vi "main.vi"() -> ()   [LabVIEW 2016]
uses:
  TypeDefs/scan_settings.ctl
  TypeDefs/State Enumerate Ring.ctl
panel:
  out "Settings folder path":path
  out "Date array":string[](array[string])
  out "Abort initalisation?":bool
  out "Scan stopped?":bool
  in  "Tab Control":T1(tab)
  in  "Manual mode":bool
  in  "Load details from file":bool
  in  "Save details to file":bool
  out "Keithley SMU":bool
  in  "User Name":string
  in  "Exeriment Title":string
  out "Status:":string
  in  "Device details":T2={"Cell Position"=1, "Cell Label"="", "Pixel to measure"=0, "Area (cm^2)"=0.0919, "Variable"="", "Variable value"="", "Scan settings"=0} {"Scan settings" items=["Default_inv"]; "Pixel to measure" items=["All", "1", "2", "3", "4", "5", "6", "7", "8"]}
  in  "Scan settings":T3={"J-V scan"=TRUE, "Start voltage (V)"=0.0, "End voltage (V)"=1.4, "Step voltage (V)"=0.01, "Scan both directions"=TRUE, "Inverted device structure"=FALSE, "Settling delay (ms)"=10.0, "Measurement speed"=0, "Scan rate (V/s)"=1.0, "Stabilisation time (s)"=0.0, "Stabilisation mode"=0, "Stabilisation value (V or A) "=0.0, "Illumination"=2, "Stabilisation in the dark?"=FALSE, "Repeat light scans"=FALSE, "No. of repeat scans"=2.0, "Only repeat for best pixel"=7, "J-t scan"=FALSE, "J-t best pixel only"=7, "J-t start voltage (V)"=0.0, "J-t end voltage (V)"=1.4, "J-t step voltage (V)"=0.01, "Step time (s)"=1.0, "J-t scan both directions"=TRUE, "J-t inverted device structure"=FALSE, "J-t settling delay (ms)"=0.0, "J-t measurement speed"=0, "J-t illumination"=1, "Max. power stabilisation"=FALSE, "Max power best pixel only"=7, "Max. power point tracker"=FALSE, "Vmp from J-V scan"=FALSE, "Max P stab. Specific voltage"=FALSE, "Vmp (V)"=0.7, "Stabilisation time step (s)"=1.0, "Total stabilisation time (s)"=100.0} {"J-t settling delay (ms)" min=10.0; "J-t illumination" items=["Light only", "Dark only", "Light then dark", "Dark then light"]; "Measurement speed" items=["Fast", "Normal", "High accuracy"]; "Illumination" items=["Light only", "Dark only", "Light then dark", "Dark then light"]; "Only repeat for best pixel" items=["only for best pixel", "for best 2 pixels", "for best 3 pixels", "for best 4 pixels", "for best 5 pixels", "for best 6 pixels", "for best 7 pixels", "for all pixels"]; "No. of repeat scans" min=1.0 step=1.0; "Max power best pixel only" items=["only the best pixel", "the best 2 pixels", "the best 3 pixels", "the best 4 pixels", "the best 5 pixels", "the best 6 pixels", "the best 7 pixels", "all pixels"]; "J-t best pixel only" items=["only the best pixel", "the best 2 pixels", "the best 3 pixels", "the best 4 pixels", "the best 5 pixels", "the best 6 pixels", "the best 7 pixels", "all pixels"]; "J-t measurement speed" items=["Fast", "Normal", "High Accuracy"]; "Stabilisation mode" items=["V", "I"]; "Settling delay (ms)" min=10.0}
  in  "Delete settings":bool
  in  "Save new settings":bool
  in  "Check Saved Settings":u16(ring) items=["Default_inv"]
  in  "Save New Settings As...":string
  in  "Update":bool
  in  "Exit":bool
  out "QuickMUX":bool
  in  "Lamp off":bool=TRUE
  out "Measurement status:":string
  out "Log Table":string[][](table)
  out "JV Curve":cluster{"Y":dbl[], "Y":dbl[]}[](graph)
  in  "Stop Scan 2":bool
  in  "Start Scan":bool
  in  "Generate report":bool
  out "Current (A)":dbl
  in  "Pixel":i64=1 min=1 max=8 step=1
  in  "error in (no error) 3":errorcluster
  in  "Change pin on pcb":bool
  in  "Measure current":bool
  out "File path for master log":path
  out "VISA resource name":refnum<visa-resource-name>="GPIB1::24::INSTR"
  # "Connected instruments"
  # "Label"
  # "Pixel"
  # "Condition"
  # "Jsc"
  # "Voc"
  # "PCE"
  # "FF"
  # "Vmp"
  # "Pixel Selection"
  # "Current Measurement"
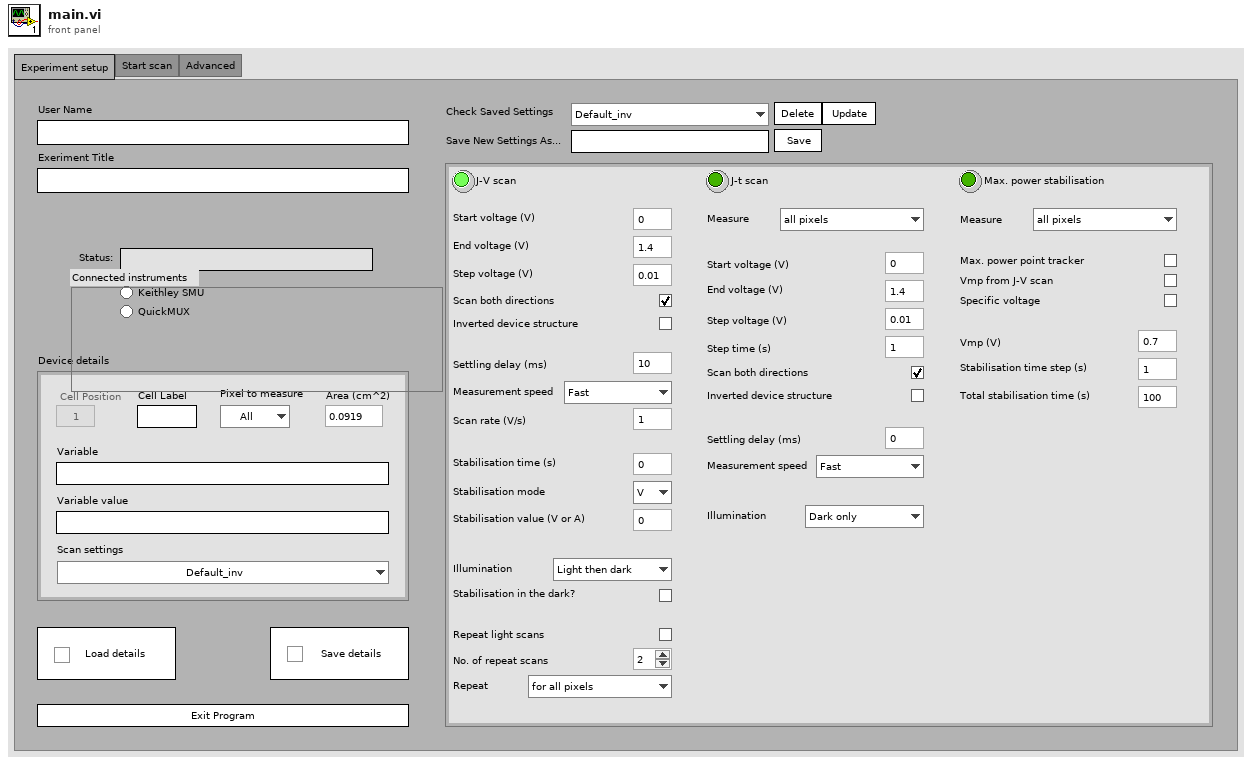
[diagram p1: front panel]
types:
  T1 = enum32{"Experiment setup", "Start scan", "Advanced"}
  T2 = cluster{"Cell Position":i32, "Cell Label":string, "Pixel to measure":u16, "Area (cm^2)":dbl, "Variable":string, "Variable value":string, "Scan settings":u16}
  T3 = typedef "scan_settings.ctl" = cluster{"J-V scan":bool, "Start voltage (V)":dbl, "End voltage (V)":dbl, "Step voltage (V)":dbl, "Scan both directions":bool, "Inverted device structure":bool, "Settling delay (ms)":dbl, "Measurement speed":u8, "Scan rate (V/s)":dbl, "Stabilisation time (s)":dbl, "Stabilisation mode":u16, "Stabilisation value (V or A) ":dbl, "Illumination":u16, "Stabilisation in the dark?":bool, "Repeat light scans":bool, "No. of repeat scans":dbl, "Only repeat for best pixel":u16, "J-t scan":bool, "J-t best pixel only":u16, "J-t start voltage (V)":dbl, "J-t end voltage (V)":dbl, "J-t step voltage (V)":dbl, "Step time (s)":dbl, "J-t scan both directions":bool, "J-t inverted device structure":bool, "J-t settling delay (ms)":dbl, "J-t measurement speed":u16, "J-t illumination":u16, "Max. power stabilisation":bool, "Max power best pixel only":u16, "Max. power point tracker":bool, "Vmp from J-V scan":bool, "Max P stab. Specific voltage":bool, "Vmp (V)":dbl, "Stabilisation time step (s)":dbl, "Total stabilisation time (s)":dbl}
  T4 = typedef "State Enumerate Ring.ctl" = enum16{"Initialise", "Idle", "Measure", "Notify"}
  T5 = enum8{"Enabled", "Disabled", "Disabled and Grayed Out"}
  T6 = cluster{"Cell Position":i32, "Cell Label":string, "Pixel to measure":u16, "Area (cm^2)":dbl, "Variable":string, "Variable value":string, "Scan settings in queue":u16, "Light or dark":string, "Measurement type":string}[]
  T7 = cluster{"Cell Position":i32, "Cell Label":string, "Pixel to measure":u16, "Area (cm^2)":dbl, "Variable":string, "Variable value":string, "Scan settings in queue":u16, "Light or dark":string, "Measurement type":string}
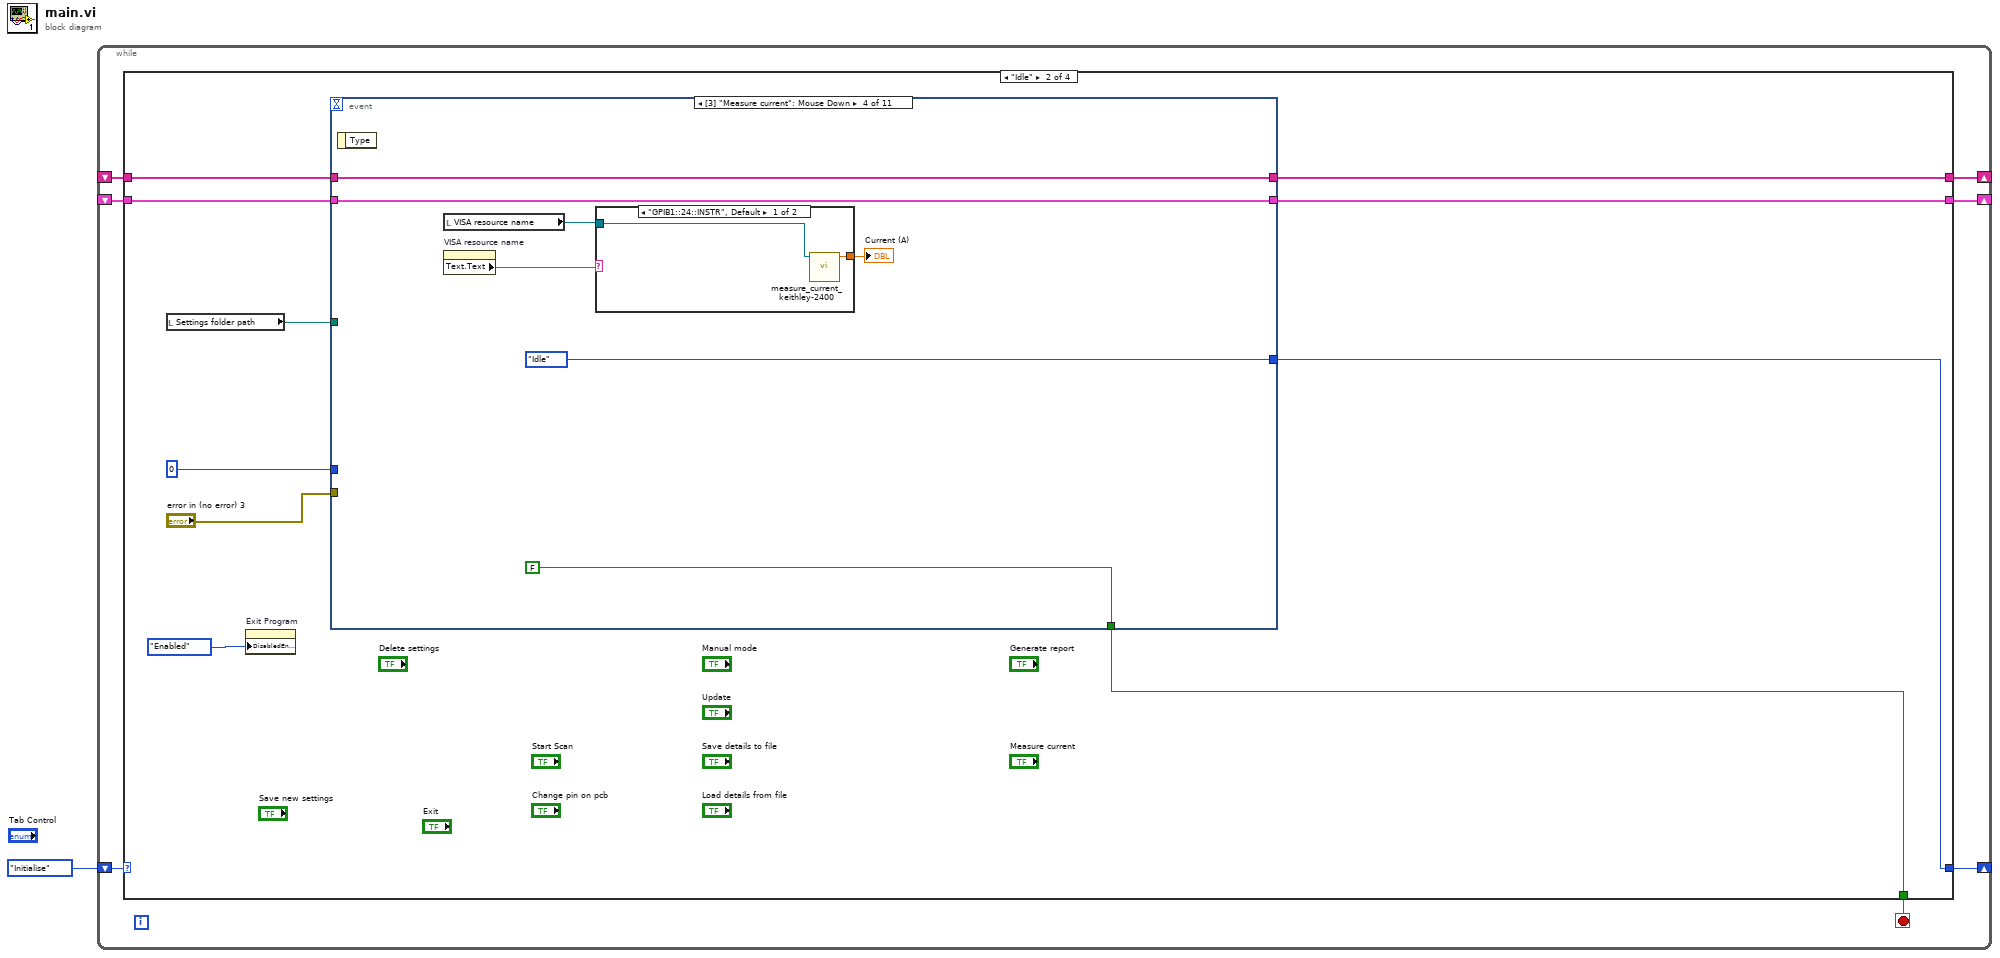
[diagram p0: block diagram]
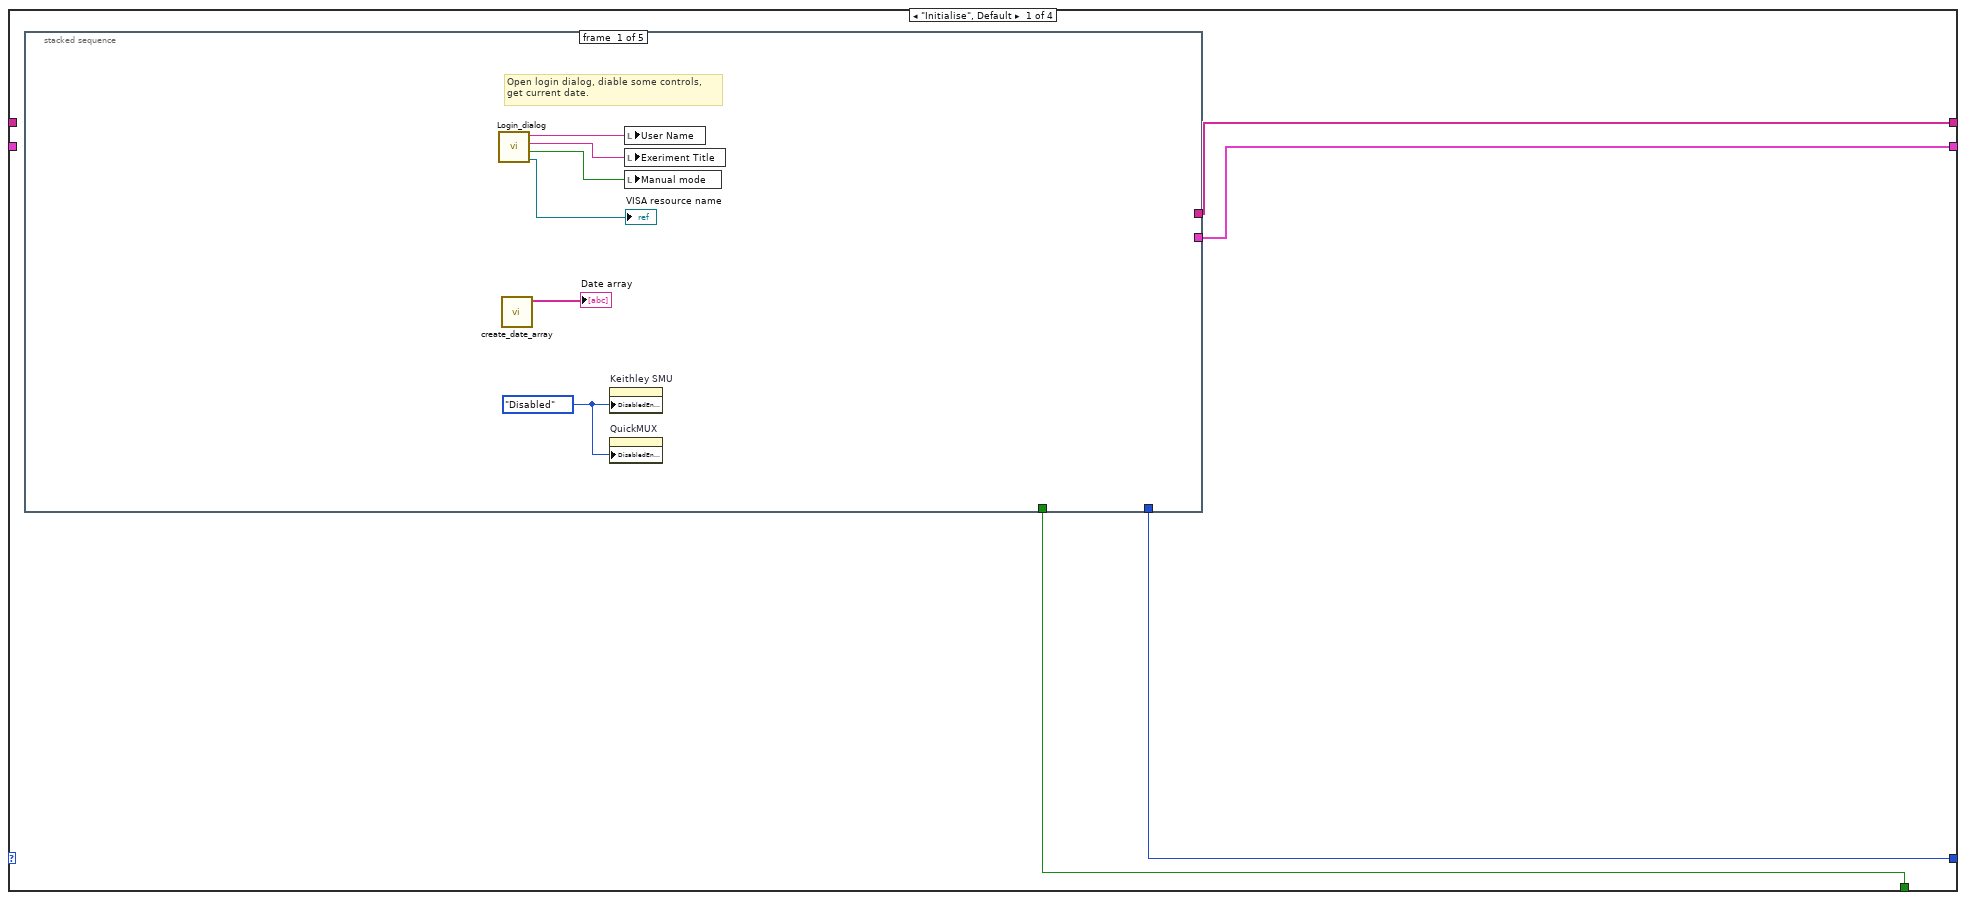
[diagram p2: hidden frame]
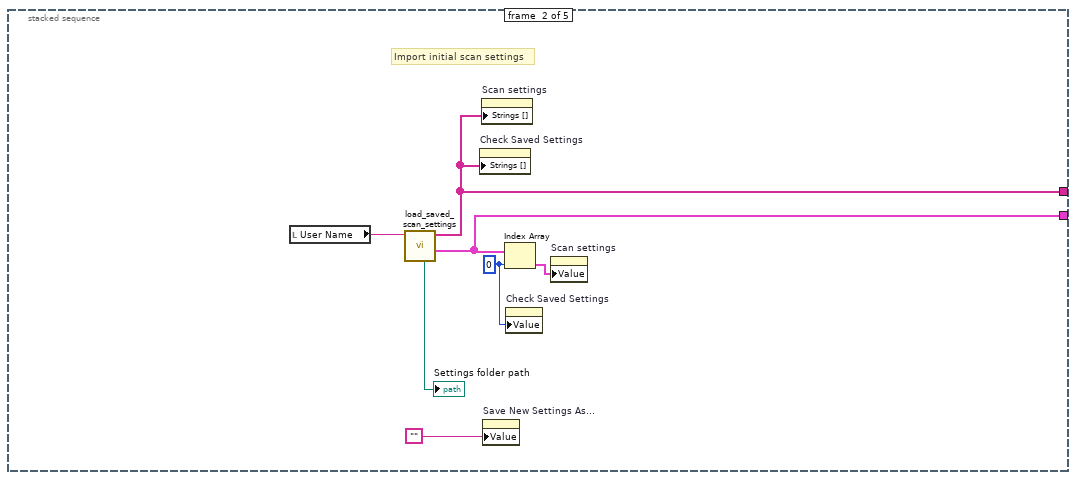
[diagram p3: hidden frame]
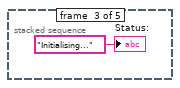
[diagram p4: hidden frame]
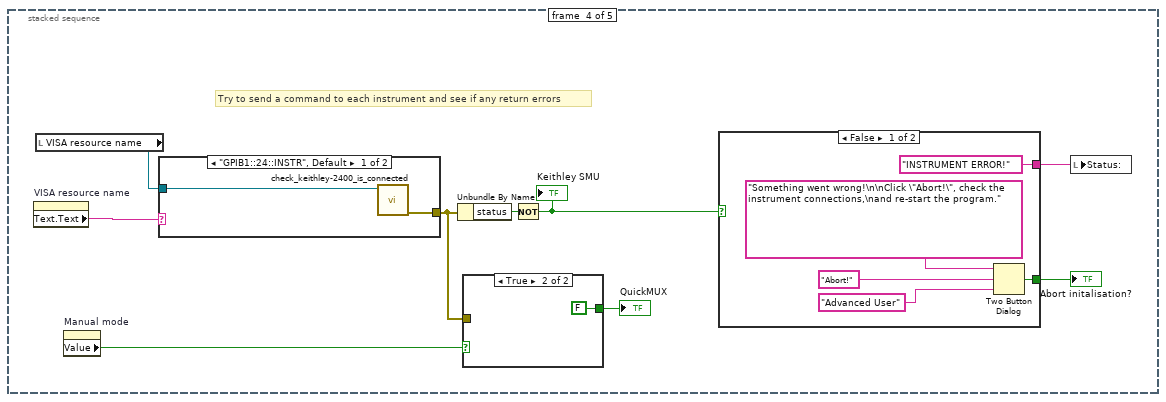
[diagram p5: hidden frame]
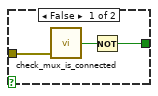
[diagram p6: hidden frame]
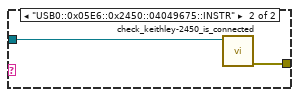
[diagram p7: hidden frame]
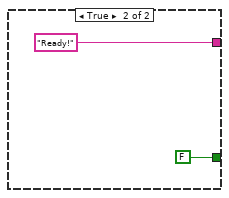
[diagram p8: hidden frame]
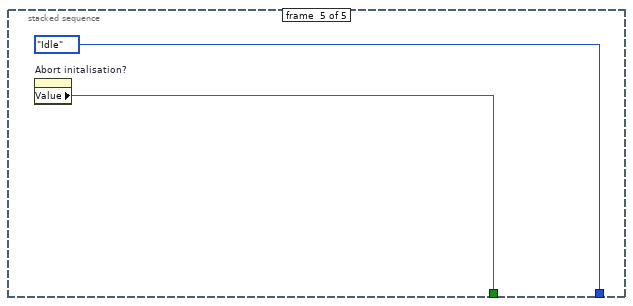
[diagram p9: hidden frame]
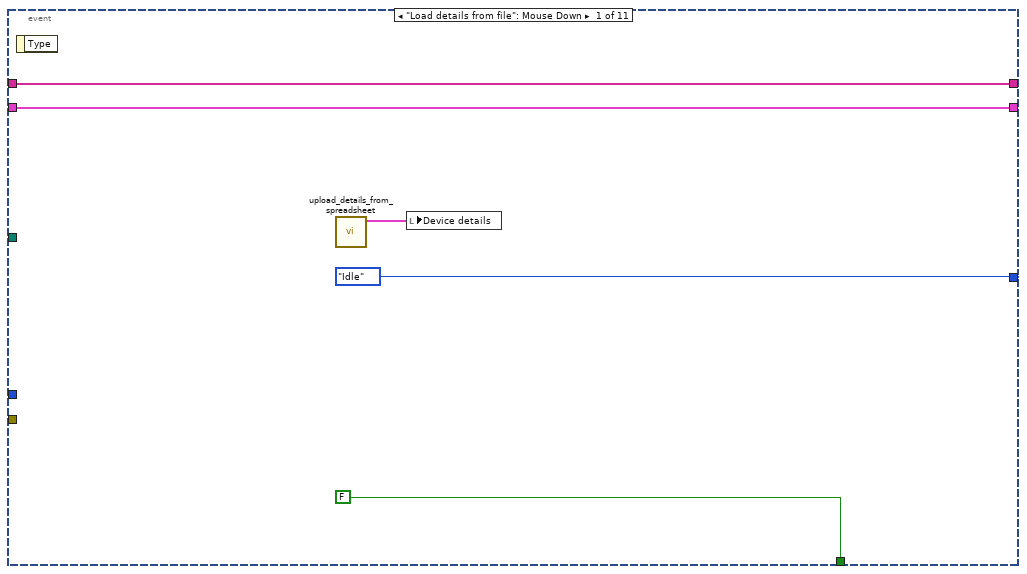
[diagram p10: hidden frame]
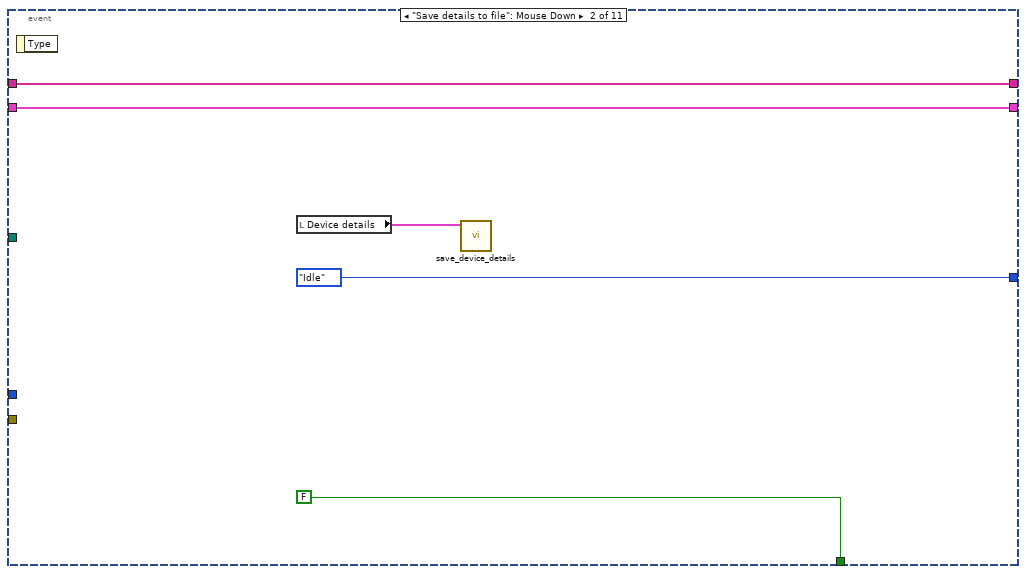
[diagram p11: hidden frame]
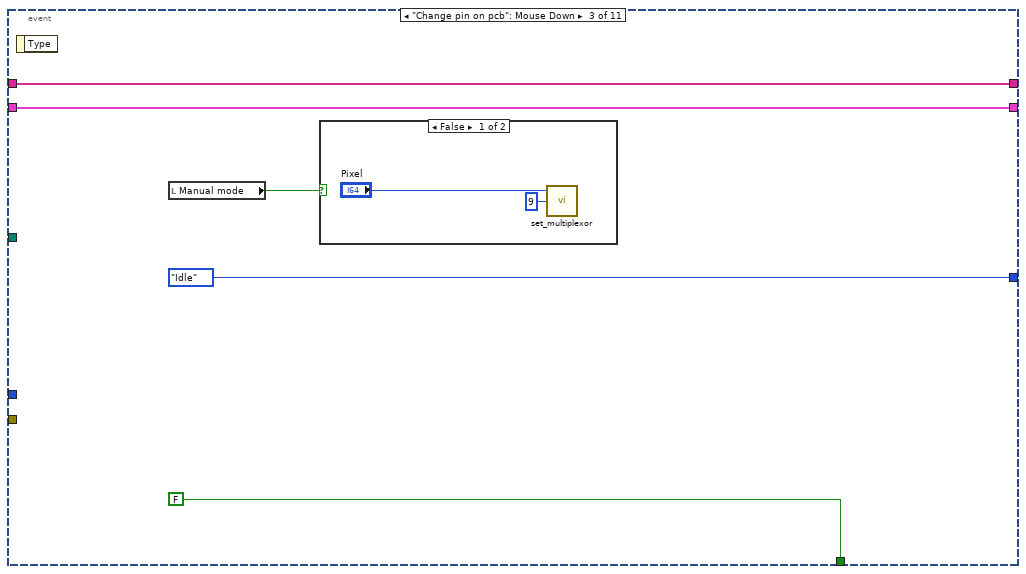
[diagram p12: hidden frame]
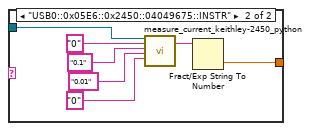
[diagram p14: hidden frame]
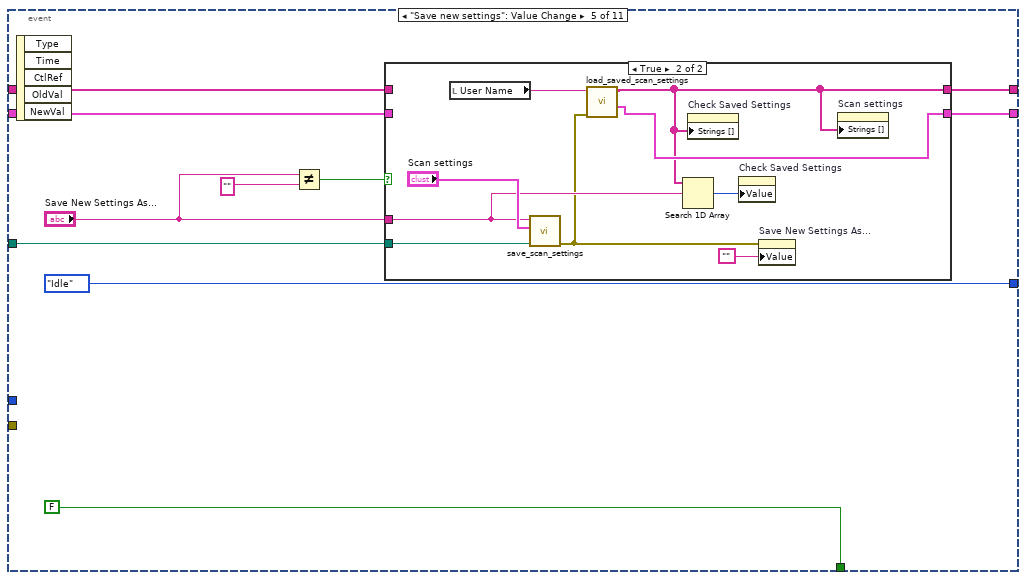
[diagram p15: hidden frame]
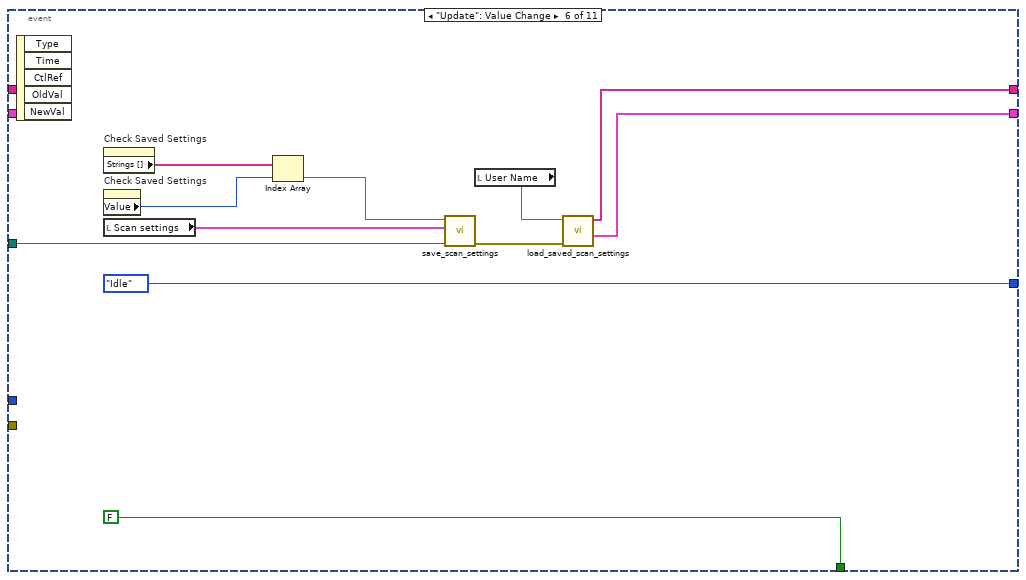
[diagram p17: hidden frame]
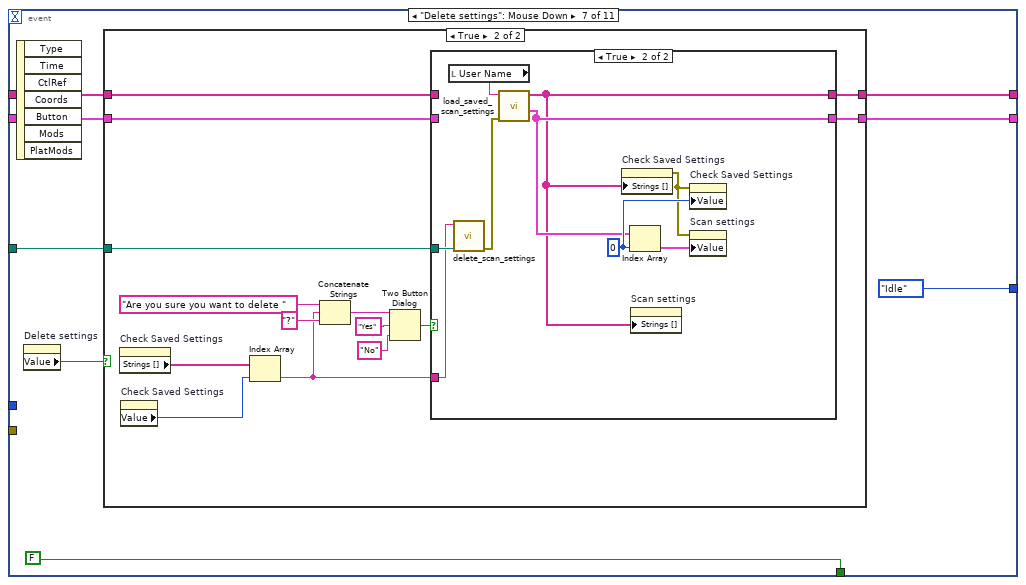
[diagram p18: hidden frame]
diagram:
  n1 = while {
    shift-right: [w3] -> _
    shift-left: _ -> [w5]
    shift-right: [w4] -> _
    shift-left: _ -> [w6]
    shift-right: [w7] -> _
    shift-left: State_Enumerate_Ring."Initialise" ("Enum") -> [w8]
    stop <- w2 stop-if-true
    n2 = case shown="\"Idle\"" w8 {
      tunnel: [w12 w53 State_Enumerate_Ring."Notify" ("Enum") w413] -> w7
      tunnel: w6 -> [_ w60 w193 w417]
      tunnel: w5 -> [_ w59 w190 w416]
      tunnel: [w10 w58 w193 w417] -> w4
      tunnel: [w9 w57 w190 w416] -> w3
      tunnel: [w11 w55 FALSE ("Value") FALSE ("Value")] -> w2
      frame "Initialise", Default {
        n3 = stacked-sequence {
          tunnel: [_ _ _ _ State_Enumerate_Ring."Idle" ("Enum")] -> w12
          tunnel: [_ _ _ _ w51] -> w11
          tunnel: [_ w24 _ _ _] -> w10
          tunnel: [_ w23 _ _ _] -> w9
          frame #0 {
            w13 = T5."Disabled" ("Disabled")
            # "Open login dialog, diable some controls,\nget current date."
            n4 = call "Login_dialog.vi"() -> ("VISA resource name"=→"VISA resource name":refnum<visa-resource-name>, "Manual mode out"=w15:bool, "Experiment title out"=w16:string, "User name out"=w17:string)  [unwired: 8 in]
            n5 = call "create_date_array.vi"() -> ("Date Array"=→"Date array":string[])  [unwired: 11 in]
            n6 = property on="Keithley SMU" class="Bool (strict)"("DisabledEnum"=w13) -> ()  [unwired: 2 in, 2 out]
            n7 = property on="QuickMUX" class="Bool (strict)"("DisabledEnum"=w13) -> ()  [unwired: 2 in, 2 out]
            n8 = local write "User Name"(w17) -> ()
            n9 = local write "Exeriment Title"(w16) -> ()
            n10 = local write "Manual mode"(w15) -> ()
          }
          frame #1 {
            w21 = 0 ("index")
            # "Import initial scan settings"
            n11 = local read "User Name"() -> (w19:string)
            n12 = call "load_saved_scan_settings.vi"("User name"=w19) -> ("Scan settings array"=w23:T3[], "Scan settings name array"=w24:string[], "Settings folder path"=→"Settings folder path":path)  [unwired: 7 in, 1 out]
            n13 = property on="Check Saved Settings" class="Ring (strict)"("Strings []"=w24) -> ()  [unwired: 2 in, 2 out]
            n14 = property on="Scan settings" class="Ring (strict)"("Strings []"=w24) -> ()  [unwired: 2 in, 2 out]
            n15 = property on="Save New Settings As..." class="Str"("Value"="") -> ()  [unwired: 2 in, 2 out]
            n16 = Index Array(array=w23, index=w21) -> (element=w22:T3)
            n17 = property on="Check Saved Settings" class="Ring (strict)"("Value"=w21) -> ()  [unwired: 2 in, 2 out]
            n18 = property on="Scan settings" class="Clust (strict)"("Value"=w22) -> ()  [unwired: 2 in, 2 out]
          }
          frame #2 {
            "Status:" <- "Initialising..." ("Instrument status")
          }
          frame #3 {
            # "Try to send a command to each instrument and see if any return errors"
            n19 = property on="VISA resource name" class="VISAName"() -> ("Text.Text"=w29:string)  [unwired: 2 in, 2 out]
            n20 = local read "VISA resource name"() -> (w28:refnum<visa-resource-name>)
            n21 = property on="Manual mode" class="Bool (strict)"() -> ("Value"=w27:bool)  [unwired: 2 in, 2 out]
            n22 = case shown="\"GPIB1::24::INSTR\", Default" w29 {
              tunnel: [w41 w43] -> w31
              tunnel: w28 -> [w40 w42]
              frame "GPIB1::24::INSTR", Default {
                n23 = call "check_keithley-2400_is_connected.vi"("VISA resource name"=w40) -> ("error out"=w41:errorcluster)  [unwired: 10 in]
              }
              frame "USB0::0x05E6::0x2450::04049675::INSTR" {
                n24 = call "check_keithley-2450_is_connected.vi"("VISA resource name"=w42) -> ("error out"=w43:errorcluster)  [unwired: 10 in]
              }
            }
            n25 = Unbundle By Name(w31) -> ("status"=w34:bool)
            n26 = case shown="True" w27 {
              tunnel: w31 -> [w38 _]
              tunnel: [w37 FALSE] -> w30
              frame False {
                n27 = call "check_mux_is_connected.vi"("error in (no error)"=w38) -> ("error?"=w36:bool)  [unwired: 4 in]
                n28 = Not(x=w36) -> (.not. x?=w37:bool)
              }
              frame True {
              }
            }
            "QuickMUX" <- w30
            n29 = Not(x=w34) -> (.not. x?=w32:bool)
            "Keithley SMU" <- w32
            n30 = case shown="False" w32 {
              tunnel: ["INSTRUMENT ERROR!" ("Instrument status") "Ready!" ("Instrument status")] -> w35
              tunnel: [w46 FALSE ("T button?")] -> w33
              frame False {
                n31 = Two Button Dialog(message="Something went wrong!\n\nClick \"Abort!\", check the instrument connections,\nand re-start the program.", 1:"Advanced User" ("T button name (\"OK\")"), 2:"Abort!" ("F button name (\"Cancel\")")) -> (T button?=w46:bool)
              }
              frame True {
              }
            }
            "Abort initalisation?" <- w33
            n32 = local write "Status:"(w35) -> ()
          }
          frame #4 {
            n33 = property on="Abort initalisation?" class="Bool (strict)"() -> ("Value"=w51:bool)  [unwired: 2 in, 2 out]
          }
        }
      }
      frame "Idle" {
        n34 = local read "Settings folder path"() -> (w54:path)
        n35 = property on="Exit Program" class="Bool (strict)"("DisabledEnum"=T5."Enabled" ("Disabled")) -> ()  [unwired: 2 in, 2 out]
        n36 = event shown="[3] \"Measure current\": Mouse Down" {
          selector: _ -> [_ _ _ _ _ _ _ _ _ _ _]
          dyn-events: _ -> [_ _ _ _ _ _ _ _ _ _ _]
          timeout: _ -> [_ _ _ _ _ _ _ _ _ _ _]
          tunnel: 0 -> [_ _ _ _ _ _ _ _ _ _ _]
          tunnel: "error in (no error) 3" -> [_ _ _ _ _ _ _ _ _ _ _]
          tunnel: w60 -> [w66 w71 w76 w84 w99 _ w134 w167 w170 w181 w186]
          tunnel: w59 -> [w65 w70 w75 w83 w98 _ w135 w166 w169 w180 w185]
          tunnel: w54 -> [_ _ _ _ w103 w123 w131 _ _ _ _]
          tunnel: [w66 w71 w76 w84 w102 w119 w133 w167 w170 w181 w186] -> w58
          tunnel: [w65 w70 w75 w83 w101 w118 w132 w166 w169 w180 w185] -> w57
          tunnel: [State_Enumerate_Ring."Idle" ("Enum") State_Enumerate_Ring."Idle" ("Enum") State_Enumerate_Ring."Idle" ("Enum") State_Enumerate_Ring."Idle" ("Enum") State_Enumerate_Ring."Idle" ("Enum") State_Enumerate_Ring."Idle" ("Enum") State_Enumerate_Ring."Idle" ("Enum") State_Enumerate_Ring."Idle" ("Enum") State_Enumerate_Ring."Idle" ("Enum") State_Enumerate_Ring."Measure" ("Enum") State_Enumerate_Ring."Idle" ("Enum")] -> w53
          tunnel: [FALSE ("Value") FALSE ("Value") FALSE ("Value") FALSE ("Value") FALSE ("Value") FALSE ("Value") FALSE ("Value") FALSE ("Value") FALSE ("Value") FALSE ("Value") w183] -> w55
          event "Load details from file": Mouse Down {
            n37 = event-data() -> ()  [unwired: 1 in, 1 out]
            n38 = call "upload_details_from_spreadsheet.vi"() -> ("Device details"=w63:T2)  [unwired: 11 in]
            n39 = local write "Device details"(w63) -> ()
          }
          event "Save details to file": Mouse Down {
            n40 = event-data() -> ()  [unwired: 1 in, 1 out]
            n41 = local read "Device details"() -> (w68:T2)
            n42 = call "save_device_details.vi"("Device details"=w68) -> ()  [unwired: 11 in]
          }
          event "Change pin on pcb": Mouse Down {
            n43 = event-data() -> ()  [unwired: 1 in, 1 out]
            n44 = local read "Manual mode"() -> (w73:bool)
            n45 = case shown="False" w73 {
              frame False {
                n46 = call "set_multiplexor.vi"("Common Input Channel"=u16 9, "Pixel Input Channel"="Pixel") -> ()  [unwired: 3 in, 1 out]
              }
              frame True {
              }
            }
          }
          event "Measure current": Mouse Down {
            n47 = event-data() -> ()  [unwired: 1 in, 1 out]
            n48 = local read "VISA resource name"() -> (w81:refnum<visa-resource-name>)
            n49 = property on="VISA resource name" class="VISAName"() -> ("Text.Text"=w80:string)  [unwired: 2 in, 2 out]
            n50 = case shown="\"GPIB1::24::INSTR\", Default" w80 {
              tunnel: [w88 w89] -> w86
              tunnel: w81 -> [w87 w95]
              frame "GPIB1::24::INSTR", Default {
                n51 = call "measure_current_keithley-2400.vi"("VISA resource name"=w87) -> ("Current"=w88:dbl)  [unwired: 9 in, 1 out]
              }
              frame "USB0::0x05E6::0x2450::04049675::INSTR" {
                n52 = call "measure_current_keithley-2450_python.vi"("VISA resource name"=w95, "voltage (V)"="0", "compliance (A)"="0.1", "nplc"="0.01", "settling delay (s)"="0") -> ("current (A)"=w90:string)  [unwired: 12 in, 2 out]
                n53 = Fract/Exp String To Number(string=w90) -> (number=w89:dbl)  [unwired: 3 in, 1 out]
              }
            }
            "Current (A)" <- w86
          }
          event "Save new settings": Value Change {
            n54 = event-data() -> ()  [unwired: 1 in, 5 out]
            n55 = Not Equal?(x="Save New Settings As...", y="") -> (x != y?=w96:bool)
            n56 = case shown="True" w96 {
              tunnel: [w106 w114] -> w101
              tunnel: [w107 w108] -> w102
              tunnel: w103 -> [_ w116]
              tunnel: "Save New Settings As..." -> [_ w113]
              tunnel: w99 -> [w107 _]
              tunnel: w98 -> [w106 _]
              frame False {
              }
              frame True {
                n57 = local read "User Name"() -> (w109:string)
                n58 = call "save_scan_settings.vi"("Path"=w116, "New scan settings"="Scan settings", "New name"=w113) -> ("error out"=w110:errorcluster)  [unwired: 8 in]
                n59 = call "load_saved_scan_settings.vi"("error in (no error)"=w110, "User name"=w109) -> ("Scan settings array"=w114:T3[], "Scan settings name array"=w108:string[])  [unwired: 6 in, 2 out]
                n60 = Search 1D Array(1D array=w108, element=w113) -> (index of element=w112:i32)  [unwired: 1 in]
                n61 = property on="Check Saved Settings" class="Ring (strict)"("Strings []"=w108) -> ()  [unwired: 2 in, 2 out]
                n62 = property on="Check Saved Settings" class="Ring (strict)"("Value"=w112) -> ()  [unwired: 2 in, 2 out]
                n63 = property on="Save New Settings As..." class="Str"(error in=w110, "Value"="") -> ()  [unwired: 1 in, 2 out]
                n64 = property on="Scan settings" class="Ring (strict)"("Strings []"=w108) -> ()  [unwired: 2 in, 2 out]
              }
            }
          }
          event "Update": Value Change {
            n65 = event-data() -> ()  [unwired: 1 in, 5 out]
            n66 = property on="Check Saved Settings" class="Ring (strict)"() -> ("Strings []"=w127:string[])  [unwired: 2 in, 2 out]
            n67 = property on="Check Saved Settings" class="Ring (strict)"() -> ("Value"=w126:u16)  [unwired: 2 in, 2 out]
            n68 = local read "Scan settings"() -> (w124:T3)
            n69 = Index Array(array=w127, index=w126) -> (element=w125:string)
            n70 = call "save_scan_settings.vi"("Path"=w123, "New scan settings"=w124, "New name"=w125) -> ("error out"=w120:errorcluster)  [unwired: 8 in]
            n71 = local read "User Name"() -> (w117:string)
            n72 = call "load_saved_scan_settings.vi"("error in (no error)"=w120, "User name"=w117) -> ("Scan settings array"=w118:T3[], "Scan settings name array"=w119:string[])  [unwired: 6 in, 2 out]
          }
          event "Delete settings": Mouse Down {
            n73 = event-data() -> ()  [unwired: 1 in, 7 out]
            n74 = property on="Delete settings" class="Bool (strict)"() -> ("Value"=w130:bool)  [unwired: 2 in, 2 out]
            n75 = case shown="True" w130 {
              tunnel: w135 -> [w136 w143]
              tunnel: w134 -> [w137 w142]
              tunnel: [w137 w141] -> w133
              tunnel: [w136 w140] -> w132
              tunnel: w131 -> [_ w139]
              frame False {
              }
              frame True {
                n76 = property on="Check Saved Settings" class="Ring (strict)"() -> ("Strings []"=w149:string[])  [unwired: 2 in, 2 out]
                n77 = property on="Check Saved Settings" class="Ring (strict)"() -> ("Value"=w148:u16)  [unwired: 2 in, 2 out]
                n78 = Index Array(array=w149, index=w148) -> (element=w138:string)
                n79 = Concatenate Strings("Are you sure you want to delete " ("string"), w138, "?" ("string")) -> (w145:string)
                n80 = Two Button Dialog(message=w145, 1:"No" ("F button name (\"Cancel\")"), 2:"Yes" ("T button name (\"OK\")")) -> (T button?=w144:bool)
                n81 = case shown="True" w144 {
                  tunnel: w143 -> [w152 _]
                  tunnel: w142 -> [w153 _]
                  tunnel: [w153 w154] -> w141
                  tunnel: [w152 w157] -> w140
                  tunnel: w139 -> [_ w162]
                  tunnel: w138 -> [_ w161]
                  frame False {
                  }
                  frame True {
                    w159 = 0 ("index")
                    n82 = local read "User Name"() -> (w155:string)
                    n83 = call "delete_scan_settings.vi"("Path"=w162, "Scan settings name"=w161) -> ("error out"=w156:errorcluster)  [unwired: 9 in]
                    n84 = call "load_saved_scan_settings.vi"("error in (no error)"=w156, "User name"=w155) -> ("Scan settings array"=w157:T3[], "Scan settings name array"=w154:string[])  [unwired: 6 in, 2 out]
                    n85 = property on="Check Saved Settings" class="Ring (strict)"("Strings []"=w154) -> (error out=w158:errorcluster)  [unwired: 2 in, 1 out]
                    n86 = Index Array(array=w157, index=w159) -> (element=w160:T3)
                    n87 = property on="Scan settings" class="Ring (strict)"("Strings []"=w154) -> ()  [unwired: 2 in, 2 out]
                    n88 = property on="Check Saved Settings" class="Ring (strict)"(error in=w158, "Value"=w159) -> ()  [unwired: 1 in, 2 out]
                    n89 = property on="Scan settings" class="Clust (strict)"(error in=w158, "Value"=w160) -> ()  [unwired: 1 in, 2 out]
                  }
                }
              }
            }
          }
          event "Check Saved Settings": Value Change {
            n90 = event-data() -> ()  [unwired: 1 in, 1 out]
            n91 = Index Array(array=w166, index="Check Saved Settings") -> (element=w163:T3)
            n92 = property on="Scan settings" class="Clust (strict)"("Value"=w163) -> ()  [unwired: 2 in, 2 out]
          }
          event "Generate report": Value Change {
            n93 = event-data() -> ()  [unwired: 1 in, 5 out]
            n94 = flat-sequence {
              frame #0 {
                w173 = "Analysing data..." ("Status:")
                n95 = local write "Measurement status:"(w173) -> ()
                n96 = local write "Status:"(w173) -> ()
              }
              frame #1 {
                n97 = local read "File path for master log"() -> (w175:path)
                n98 = local read "Exeriment Title"() -> (w174:string)
                n99 = call "JV Data analysis from master log file.vi"("Experiment Indicator"=w174, "Master log filepath"=w175) -> ()  [unwired: 10 in]
              }
              frame #2 {
                n100 = local write "Measurement status:"("" ("Measurement status:")) -> ()
                n101 = local write "Status:"("Ready!" ("Status:")) -> ()
              }
            }
          }
          event "Start Scan": Mouse Down {
            n102 = event-data() -> ()  [unwired: 1 in, 1 out]
            n103 = local write "Status:"("Measuring" ("Status:")) -> ()
          }
          event "Exit": Mouse Down {
            n104 = event-data() -> ()  [unwired: 1 in, 7 out]
            n105 = property on="Exit" class="Bool (strict)"() -> ("Value"=w183:bool)  [unwired: 2 in, 2 out]
          }
        }
      }
      frame "Measure" {
        n106 = call "build_queue.vi"("Scan settings array"=w190, "Device details"="Device details") -> ("Measurement queue"=w189:T6)  [unwired: 9 in]
        n107 = while {
          shift-right: [w195] -> _
          shift-left: w189 -> [w201]
          tunnel: w190 -> [w196]
          stop <- w198 stop-if-true
          # "Loop over measurement queue until\nit's empty or user presses stop."
          n108 = Array Size(array=w201) -> (size(s)=w194:i32)
          n109 = Equal?(x=0, y=w194) -> (x = y?=w199:bool)
          n110 = Compound Arithmetic op=OR(w199, "Stop Scan 2") -> (w198:bool)
          "Scan stopped?" <- w198
          n111 = case shown="False" w198 {
            tunnel: [w215 w412] -> w195
            tunnel: w201 -> [w214 w412]
            tunnel: w196 -> [w213 _]
            frame False {
              n112 = Delete From Array(array=w214, index=0) -> (deleted portion=w206:T7, array with subset deleted=w215:T6)  [unwired: 1 in]
              n113 = local read "Date array"() -> (w204:string[])
              n114 = Unbundle By Name(w206) -> ("Pixel to measure"=w207:u16, "Scan settings in queue"=w203:u16, "Measurement type"=w202:string)
              n115 = call "build_meas_status_string.vi"("Cell details cluster in"=w206) -> ("Measurement status"=→"Measurement status:":string)  [unwired: 10 in]
              n116 = Index Array(array=w213, index=w203) -> (element=w211:T3)
              n117 = case shown="\"Max P Stabilization\"" w202 {
                tunnel: w206 -> [w227 w262 w324 w377]
                tunnel: "User Name" -> [w226 w261 w323 w376]
                tunnel: "Exeriment Title" -> [w225 w260 w322 w375]
                tunnel: w211 -> [w219 w259 w321 w374]
                tunnel: [w224 w267 w320 w373] -> w210
                tunnel: w207 -> [w216 w252 w311 w364]
                tunnel: w204 -> [w217 w254 w306 w360]
                frame "JV Scan", Default {
                  n118 = flat-sequence {
                    tunnel: [w230] -> w223
                    tunnel: [w233] -> w222
                    tunnel: [w232] -> w221
                    tunnel: [w231] -> w220
                    tunnel: w227 -> [w230]
                    tunnel: w226 -> [w233]
                    tunnel: w225 -> [w232]
                    tunnel: w219 -> [w231]
                    tunnel: w216 -> [w228]
                    tunnel: w223 -> [w245]
                    tunnel: w222 -> [w244]
                    tunnel: w221 -> [w243]
                    tunnel: w220 -> [w242]
                    tunnel: [w240] -> w218
                    tunnel: w217 -> [w237]
                    tunnel: [w249] -> w224
                    tunnel: w218 -> [w249]
                    frame #0 {
                      # "Switch pixel if needed"
                      n119 = property on="Manual mode" class="Bool (strict)"() -> ("Value"=w229:bool)  [unwired: 2 in, 2 out]
                      n120 = case shown="False" w229 {
                        tunnel: w228 -> [w234 _]
                        frame False {
                          n121 = call "set_multiplexor.vi"("Common Input Channel"=u16 9, "Pixel Input Channel"=w234) -> ()  [unwired: 3 in, 1 out]
                        }
                        frame True {
                        }
                      }
                    }
                    frame #1 {
                      # "Take measurement"
                      n122 = local read "VISA resource name"() -> (w236:refnum<visa-resource-name>)
                      n123 = call "measure_j-v_keithley-2400.vi"("User Name"=w244, "Cell details cluster"=w245, "Date array"=w237, "Experiment Title"=w243, "Scan settings"=w242, "VISA resource name"=w236, "Skip pixel?"=FALSE) -> ("JV Curve"=w240:cluster{"Y":dbl[], "Y":dbl[]}[], "File path for master log"=→"File path for master log":path, "Log Table"=→"Log Table":string[][])  [unwired: 6 in]
                    }
                    frame #2 {
                      # "Update graph"
                      n124 = property on="JV Curve" class="XYGraph (strict)"("YScale.NameLbl.Text"="J (mA/cm^2)" ("Y Scale.Name Label.Text")) -> ()  [unwired: 2 in, 2 out]
                      n125 = for {
                        tunnel: string[] ["Scan 1", "Scan 2"] ("Measurement queue") -> [w250] mode=indexing
                        i -> [w251]
                        n126 = property on="JV Curve" class="XYGraph (strict)"("Active Plot"=w251, "Plot.Plot Name"=w250) -> ()  [unwired: 2 in, 2 out]
                      }
                      n127 = property on="JV Curve" class="XYGraph (strict)"("XScale.NameLbl.Text"="Applied Bias (V)" ("Y Scale.Name Label.Text")) -> ()  [unwired: 2 in, 2 out]
                    }
                  }
                }
                frame "Repeat JV Scan For Best" {
                  n128 = flat-sequence {
                    tunnel: w259 -> [w278]
                    tunnel: w260 -> [w279]
                    tunnel: w261 -> [w280]
                    tunnel: w262 -> [w276]
                    tunnel: [w275] -> w266
                    tunnel: [w280] -> w265
                    tunnel: [w279] -> w264
                    tunnel: [w278] -> w263
                    tunnel: w252 -> [w272]
                    tunnel: [w274] -> w256
                    tunnel: [w273] -> w255
                    tunnel: [w272] -> w253
                    tunnel: [w284] -> w271
                    tunnel: [w287] -> w270
                    tunnel: [w286] -> w269
                    tunnel: [w285] -> w268
                    tunnel: w266 -> [w284]
                    tunnel: w265 -> [w287]
                    tunnel: w264 -> [w286]
                    tunnel: w263 -> [w285]
                    tunnel: [w283] -> w257
                    tunnel: w256 -> [w283]
                    tunnel: w255 -> [w281]
                    tunnel: w253 -> [w282]
                    tunnel: w271 -> [w298]
                    tunnel: w270 -> [w297]
                    tunnel: w269 -> [w296]
                    tunnel: w268 -> [w295]
                    tunnel: [w294] -> w258
                    tunnel: w257 -> [w292]
                    tunnel: w254 -> [w291]
                    tunnel: [w302] -> w267
                    tunnel: w258 -> [w302]
                    frame #0 {
                      # "Find best pixel if needed"
                      n129 = local read "File path for master log"() -> (w277:path)
                      n130 = property on="Manual mode" class="Bool (strict)"() -> ("Value"=w273:bool)  [unwired: 2 in, 2 out]
                      n131 = call "find_best_pixel_from_log.vi"("Manual mode?"=w273, "Cell details cluster in"=w276, "Nth best pixel"=w272, "File path of JV log"=w277) -> ("Skip pixel?"=w274:bool, "Best pixel cell details cluster"=w275:T7)  [unwired: 6 in]
                    }
                    frame #1 {
                      # "Switch pixel if needed"
                      n132 = case shown="True" w281 {
                        tunnel: w282 -> [w289 _]
                        frame False {
                          n133 = call "set_multiplexor.vi"("Common Input Channel"=u16 9, "Pixel Input Channel"=w289) -> ()  [unwired: 3 in, 1 out]
                        }
                        frame True {
                        }
                      }
                    }
                    frame #2 {
                      # "Take measurement"
                      n134 = local read "VISA resource name"() -> (w290:refnum<visa-resource-name>)
                      n135 = call "measure_j-v_keithley-2400.vi"("User Name"=w297, "Cell details cluster"=w298, "Date array"=w291, "Experiment Title"=w296, "Scan settings"=w295, "VISA resource name"=w290, "Skip pixel?"=w292) -> ("JV Curve"=w294:cluster{"Y":dbl[], "Y":dbl[]}[], "Log Table"=w293:string[][])  [unwired: 6 in, 1 out]
                      n136 = local write "Log Table"(w293) -> ()
                    }
                    frame #3 {
                      # "Update graph"
                      n137 = for {
                        tunnel: string[] ["Scan 1", "Scan 2"] ("Measurement queue") -> [w303] mode=indexing
                        i -> [w304]
                        n138 = property on="JV Curve" class="XYGraph (strict)"("Active Plot"=w304, "Plot.Plot Name"=w303) -> ()  [unwired: 2 in, 2 out]
                      }
                      n139 = property on="JV Curve" class="XYGraph (strict)"("XScale.NameLbl.Text"="Applied Bias (V)" ("Y Scale.Name Label.Text")) -> ()  [unwired: 2 in, 2 out]
                      n140 = property on="JV Curve" class="XYGraph (strict)"("YScale.NameLbl.Text"="J (mA/cm^2)" ("Y Scale.Name Label.Text")) -> ()  [unwired: 2 in, 2 out]
                    }
                  }
                }
                frame "Jt Scan" {
                  n141 = flat-sequence {
                    tunnel: w321 -> [w331]
                    tunnel: w322 -> [w332]
                    tunnel: w323 -> [w333]
                    tunnel: w324 -> [w329]
                    tunnel: [w328] -> w315
                    tunnel: [w333] -> w314
                    tunnel: [w332] -> w313
                    tunnel: [w331] -> w312
                    tunnel: w311 -> [w325]
                    tunnel: [w327] -> w308
                    tunnel: [w326] -> w307
                    tunnel: [w325] -> w305
                    tunnel: [w337] -> w319
                    tunnel: [w340] -> w318
                    tunnel: [w339] -> w317
                    tunnel: [w338] -> w316
                    tunnel: w315 -> [w337]
                    tunnel: w314 -> [w340]
                    tunnel: w313 -> [w339]
                    tunnel: w312 -> [w338]
                    tunnel: [w336] -> w309
                    tunnel: w308 -> [w336]
                    tunnel: w307 -> [w334]
                    tunnel: w305 -> [w335]
                    tunnel: w319 -> [w351]
                    tunnel: w318 -> [w350]
                    tunnel: w317 -> [w349]
                    tunnel: w316 -> [w348]
                    tunnel: [w347] -> w310
                    tunnel: w309 -> [w346]
                    tunnel: w306 -> [w345]
                    tunnel: [w355] -> w320
                    tunnel: w310 -> [w355]
                    frame #0 {
                      # "Find best pixel if needed"
                      n142 = local read "File path for master log"() -> (w330:path)
                      n143 = property on="Manual mode" class="Bool (strict)"() -> ("Value"=w326:bool)  [unwired: 2 in, 2 out]
                      n144 = call "find_best_pixel_from_log.vi"("Manual mode?"=w326, "Cell details cluster in"=w329, "Nth best pixel"=w325, "File path of JV log"=w330) -> ("Skip pixel?"=w327:bool, "Best pixel cell details cluster"=w328:T7)  [unwired: 6 in]
                    }
                    frame #1 {
                      # "Switch pixel if needed"
                      n145 = case shown="False" w334 {
                        tunnel: w335 -> [w342 _]
                        frame False {
                          n146 = call "set_multiplexor.vi"("Common Input Channel"=u16 9, "Pixel Input Channel"=w342) -> ()  [unwired: 3 in, 1 out]
                        }
                        frame True {
                        }
                      }
                    }
                    frame #2 {
                      # "Take measurement"
                      n147 = local read "VISA resource name"() -> (w343:refnum<visa-resource-name>)
                      n148 = call "measure_j-t_keithley-2450.vi"() -> ()  [unwired: 11 in, 1 out]
                      n149 = call "measure_j-t_keithley-2400.vi"("Skip pixel?"=w346, "Date array"=w345, "Scan settings"=w348, "Cell details cluster"=w351, "VISA resource name"=w343, "Intensity (no. of suns)"="1", "Experiment Title"=w349, "User Name"=w350) -> ("Jt Curve"=w347:cluster{"Y":dbl[], "Y":dbl[]}[])  [unwired: 3 in]
                    }
                    frame #3 {
                      # "Update graph"
                      n150 = for {
                        tunnel: string[] ["Scan 1", "Scan 2"] ("Measurement queue") -> [w356] mode=indexing
                        i -> [w357]
                        n151 = property on="JV Curve" class="XYGraph (strict)"("Active Plot"=w357, "Plot.Plot Name"=w356) -> ()  [unwired: 2 in, 2 out]
                      }
                      n152 = property on="JV Curve" class="XYGraph (strict)"("YScale.NameLbl.Text"="J (mA/cm^2)" ("Y Scale.Name Label.Text")) -> ()  [unwired: 2 in, 2 out]
                      n153 = property on="JV Curve" class="XYGraph (strict)"("XScale.NameLbl.Text"="Time (s)" ("Y Scale.Name Label.Text")) -> ()  [unwired: 2 in, 2 out]
                    }
                  }
                }
                frame "Max P Stabilization" {
                  n154 = flat-sequence {
                    tunnel: w374 -> [w384]
                    tunnel: w375 -> [w385]
                    tunnel: w376 -> [w386]
                    tunnel: w377 -> [w383]
                    tunnel: [w382] -> w368
                    tunnel: [w386] -> w367
                    tunnel: [w385] -> w366
                    tunnel: [w384] -> w365
                    tunnel: w364 -> [w379]
                    tunnel: [w380] -> w361
                    tunnel: [w379] -> w359
                    tunnel: [w378] -> w358
                    tunnel: [w390] -> w372
                    tunnel: [w393] -> w371
                    tunnel: [w392] -> w370
                    tunnel: [w391] -> w369
                    tunnel: w368 -> [w390]
                    tunnel: w367 -> [w393]
                    tunnel: w366 -> [w392]
                    tunnel: w365 -> [w391]
                    tunnel: [w389] -> w362
                    tunnel: w361 -> [w389]
                    tunnel: w359 -> [w388]
                    tunnel: w358 -> [w387]
                    tunnel: w372 -> [w405]
                    tunnel: w371 -> [w404]
                    tunnel: w370 -> [w403]
                    tunnel: w369 -> [w402]
                    tunnel: [w401] -> w363
                    tunnel: w362 -> [w399]
                    tunnel: w360 -> [w398]
                    tunnel: [w409] -> w373
                    tunnel: w363 -> [w409]
                    frame #0 {
                      # "Find best pixel if needed"
                      n155 = local read "File path for master log"() -> (w381:path)
                      n156 = property on="Manual mode" class="Bool (strict)"() -> ("Value"=w378:bool)  [unwired: 2 in, 2 out]
                      n157 = call "find_best_pixel_from_log.vi"("Manual mode?"=w378, "Cell details cluster in"=w383, "Nth best pixel"=w379, "File path of JV log"=w381) -> ("Skip pixel?"=w380:bool, "Best pixel cell details cluster"=w382:T7)  [unwired: 6 in]
                    }
                    frame #1 {
                      # "Switch pixel if needed"
                      n158 = case shown="False" w387 {
                        tunnel: w388 -> [w394 _]
                        frame False {
                          n159 = call "set_multiplexor.vi"("Common Input Channel"=u16 9, "Pixel Input Channel"=w394) -> ()  [unwired: 3 in, 1 out]
                        }
                        frame True {
                        }
                      }
                    }
                    frame #2 {
                      # "Take measurement"
                      n160 = local read "File path for master log"() -> (w400:path)
                      n161 = local read "VISA resource name"() -> (w396:refnum<visa-resource-name>)
                      n162 = call "measure_max_power_stabilisation_keithley-2400.vi"("User Name"=w404, "Cell details cluster"=w405, "Date array"=w398, "Experiment Title"=w403, "File path of JV log"=w400, "Intensity (no. of suns)"="1", "Scan settings"=w402, "VISA resource name"=w396, "Skip pixel?"=w399) -> ("Jt Curve"=w401:cluster{"Y":dbl[], "Y":dbl[]}[])  [unwired: 6 in]
                    }
                    frame #3 {
                      # "Update graph"
                      n163 = property on="JV Curve" class="XYGraph (strict)"("XScale.NameLbl.Text"="Time (s)" ("Y Scale.Name Label.Text")) -> ()  [unwired: 2 in, 2 out]
                      n164 = for {
                        tunnel: string[] ["|PCE (%)|", "|J (mA/cm^2)|"] ("Measurement queue") -> [w410] mode=indexing
                        i -> [w411]
                        n165 = property on="JV Curve" class="XYGraph (strict)"("Active Plot"=w411, "Plot.Plot Name"=w410) -> ()  [unwired: 2 in, 2 out]
                      }
                      n166 = property on="JV Curve" class="XYGraph (strict)"("YScale.NameLbl.Text"="|PCE (%)| or |J (mA/cm^2)|" ("Y Scale.Name Label.Text")) -> ()  [unwired: 2 in, 2 out]
                    }
                  }
                }
              }
              "JV Curve" <- w210
            }
            frame True {
            }
          }
        }
        n167 = property on="Exit program" class="Bool (strict)"("DisabledEnum"=T5."Disabled and Grayed Out" ("Disabled")) -> ()  [unwired: 2 in, 2 out]
      }
      frame "Notify" {
        n168 = property on="Manual mode" class="Bool (strict)"() -> ("Value"=w414:bool)  [unwired: 2 in, 2 out]
        n169 = case shown="True" w414 {
          tunnel: [w418 State_Enumerate_Ring."Idle" ("Enum")] -> w413
          frame False {
            n170 = flat-sequence {
              tunnel: [State_Enumerate_Ring."Idle" ("Enum")] -> w418
              frame #0 {
                w419 = "Analysing data..." ("Status:")
                n171 = local write "Measurement status:"(w419) -> ()
                n172 = local write "Status:"(w419) -> ()
              }
              frame #1 {
                n173 = case shown="True" "Lamp off" {
                  frame False {
                  }
                  frame True {
                    n174 = call "Send_lamp_power_supply_command.vi"("write buffer"="STOP", "VISA resource name"=refnum<visa-resource-name> "COM10") -> ()  [unwired: 10 in]
                    n175 = call "Send_lamp_power_supply_command.vi"("write buffer"="STOP", "VISA resource name"=refnum<visa-resource-name> "COM11") -> ()  [unwired: 10 in]
                  }
                }
              }
              frame #2 {
                n176 = local write "Measurement status:"("") -> ()
                n177 = local write "Status:"("Ready!" ("Status:")) -> ()
              }
              frame #3 {
                n178 = One Button Dialog(message="Experiment complete!") -> ()  [unwired: 1 in, 1 out]
              }
              frame #4 {
              }
            }
          }
          frame True {
            n179 = local write "Status:"("Ready!" ("Status:")) -> ()
            n180 = local write "Measurement status:"("Measurement complete!" ("Measurement status:")) -> ()
          }
        }
      }
    }
  }
